vi "Exercise 7.1_Instant_Stop.vi"() -> ()   [LabVIEW 2020]
uses:
  7.1 States.ctl
panel:
  in  "Stop":bool
  out "Walk Sign":bool
  out "Green":bool
  out "Yellow":bool
  out "Red":bool
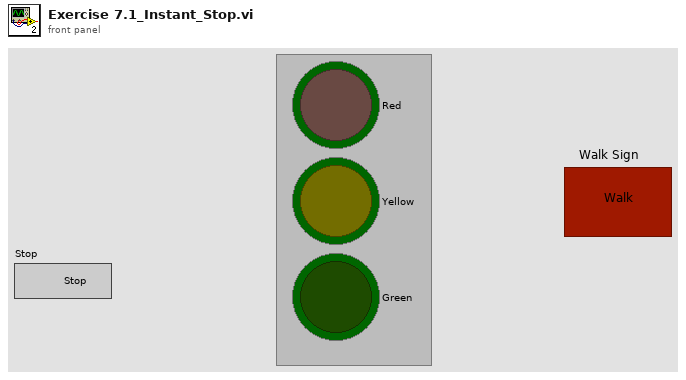
[diagram p1: front panel]
types:
  T1 = typedef "7.1 States.ctl" = enum16{"Initialize", "Green", "Yellow", "Red 1", "Red 2", "Stop"}
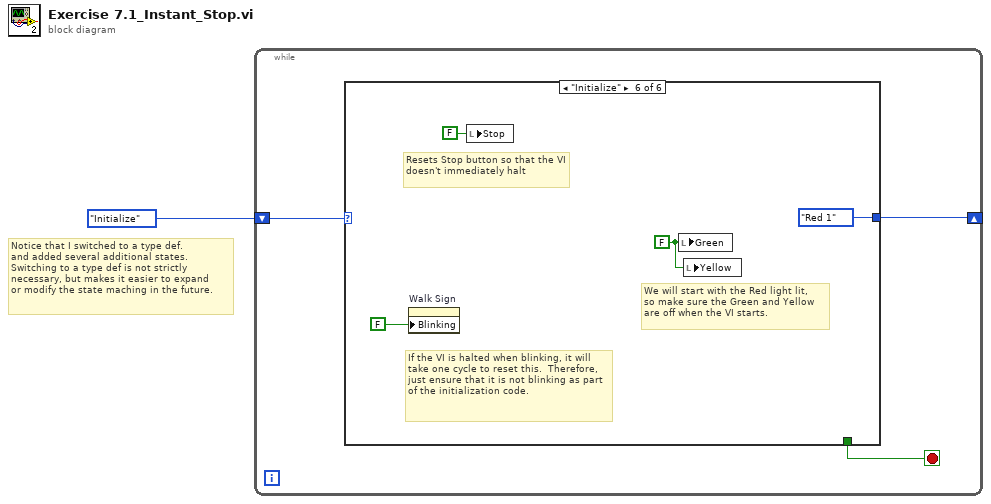
[diagram p0: block diagram]
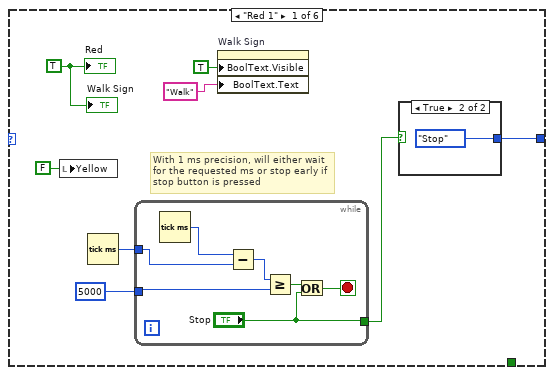
[diagram p2: hidden frame]
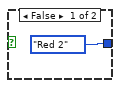
[diagram p3: hidden frame]
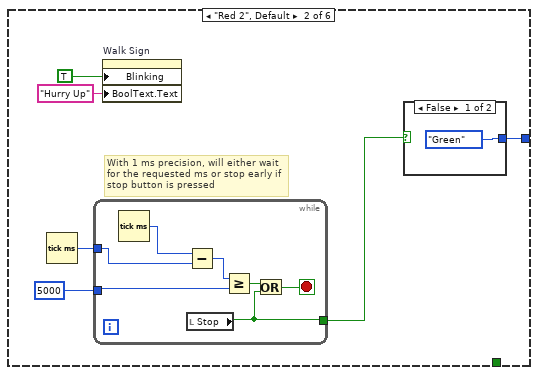
[diagram p4: hidden frame]
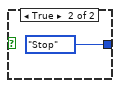
[diagram p5: hidden frame]
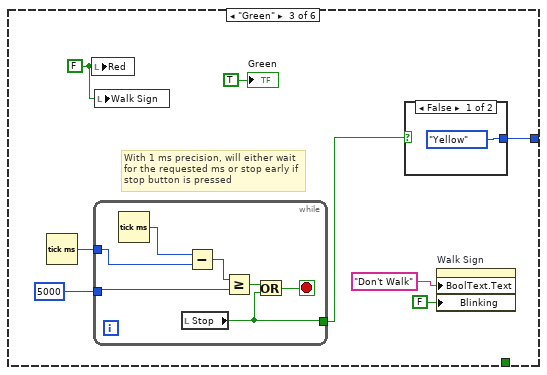
[diagram p6: hidden frame]
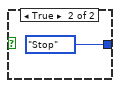
[diagram p7: hidden frame]
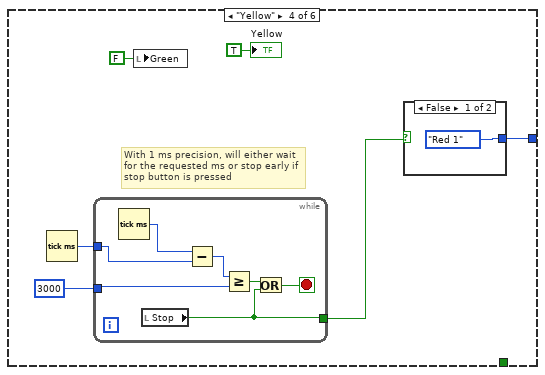
[diagram p8: hidden frame]
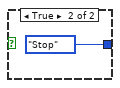
[diagram p9: hidden frame]
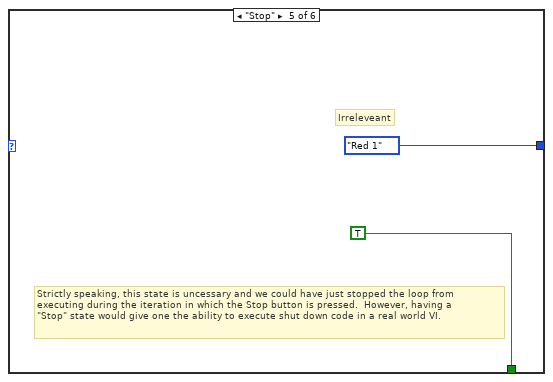
[diagram p10: hidden frame]
diagram:
  # "Notice that I switched to a type def.\nand added several additional states.\nSwitching to a type def is not strictly \nnecessary, but makes it easier to expand\nor modify the state maching in the future."
  n1 = while {
    shift-right: [w3] -> _
    shift-left: 7.1_States."Initialize" -> [w4]
    stop <- w2 stop-if-true
    n2 = case shown="\"Initialize\"" w4 {
      tunnel: [w9 w26 w41 w57 7.1_States."Red 1" 7.1_States."Red 1"] -> w3
      tunnel: [_ _ _ _ TRUE _] -> w2
      frame "Red 1" {
        w11 = TRUE ("Red")
        # "With 1 ms precision, will either wait for the requested ms or stop early if stop button is pressed"
        n3 = local write "Yellow"(FALSE ("Yellow")) -> ()
        n4 = Tick Count (ms)() -> (millisecond timer value=w7:u32)
        n5 = while {
          tunnel: w7 -> [w18]
          tunnel: u32 5000 ("milliseconds to wait") -> [w16]
          tunnel: ["Stop"] -> w5
          stop <- w14 stop-if-true
          n6 = Tick Count (ms)() -> (millisecond timer value=w19:u32)
          n7 = Subtract(x=w19, y=w18) -> (x-y=w17:u32)
          n8 = Greater Or Equal?(x=w17, y=w16) -> (x >= y?=w15:bool)
          n9 = Or(x=w15, y="Stop") -> (x .or. y?=w14:bool)
        }
        n10 = property on="Walk Sign" class="Bool"("BoolText.Visible"=TRUE ("Boolean Text.Visible"), "BoolText.Text"="Walk" ("Boolean Text.Text")) -> ()  [unwired: 2 in, 2 out]
        n11 = case shown="True" w5 {
          tunnel: [7.1_States."Red 2" 7.1_States."Stop"] -> w9
          frame False {
          }
          frame True {
          }
        }
        "Red" <- w11
        "Walk Sign" <- w11
      }
      frame "Red 2", Default {
        # "With 1 ms precision, will either wait for the requested ms or stop early if stop button is pressed"
        n12 = Tick Count (ms)() -> (millisecond timer value=w24:u32)
        n13 = while {
          tunnel: w24 -> [w33]
          tunnel: u32 5000 ("milliseconds to wait") -> [w31]
          tunnel: [w28] -> w22
          stop <- w29 stop-if-true
          n14 = Tick Count (ms)() -> (millisecond timer value=w34:u32)
          n15 = Subtract(x=w34, y=w33) -> (x-y=w32:u32)
          n16 = local read "Stop"() -> (w28:bool)
          n17 = Greater Or Equal?(x=w32, y=w31) -> (x >= y?=w30:bool)
          n18 = Or(x=w30, y=w28) -> (x .or. y?=w29:bool)
        }
        n19 = property on="Walk Sign" class="Bool"("Blinking"=TRUE, "BoolText.Text"="Hurry Up" ("Boolean Text.Text")) -> ()  [unwired: 2 in, 2 out]
        n20 = case shown="False" w22 {
          tunnel: [7.1_States."Green" 7.1_States."Stop"] -> w26
          frame False {
          }
          frame True {
          }
        }
      }
      frame "Green" {
        w44 = FALSE ("Red")
        # "With 1 ms precision, will either wait for the requested ms or stop early if stop button is pressed"
        n21 = Tick Count (ms)() -> (millisecond timer value=w39:u32)
        n22 = local write "Red"(w44) -> ()
        n23 = while {
          tunnel: w39 -> [w50]
          tunnel: u32 5000 ("milliseconds to wait") -> [w48]
          tunnel: [w45] -> w37
          stop <- w46 stop-if-true
          n24 = Tick Count (ms)() -> (millisecond timer value=w51:u32)
          n25 = local read "Stop"() -> (w45:bool)
          n26 = Subtract(x=w51, y=w50) -> (x-y=w49:u32)
          n27 = Greater Or Equal?(x=w49, y=w48) -> (x >= y?=w47:bool)
          n28 = Or(x=w47, y=w45) -> (x .or. y?=w46:bool)
        }
        n29 = local write "Walk Sign"(w44) -> ()
        n30 = case shown="False" w37 {
          tunnel: [7.1_States."Yellow" 7.1_States."Stop"] -> w41
          frame False {
          }
          frame True {
          }
        }
        n31 = property on="Walk Sign" class="Bool"("BoolText.Text"="Don't Walk" ("Boolean Text.Text"), "Blinking"=FALSE) -> ()  [unwired: 2 in, 2 out]
        "Green" <- TRUE ("Green")
      }
      frame "Yellow" {
        # "With 1 ms precision, will either wait for the requested ms or stop early if stop button is pressed"
        n32 = Tick Count (ms)() -> (millisecond timer value=w56:u32)
        n33 = while {
          tunnel: w56 -> [w65]
          tunnel: u32 3000 ("milliseconds to wait") -> [w63]
          tunnel: [w60] -> w54
          stop <- w61 stop-if-true
          n34 = Tick Count (ms)() -> (millisecond timer value=w66:u32)
          n35 = local read "Stop"() -> (w60:bool)
          n36 = Subtract(x=w66, y=w65) -> (x-y=w64:u32)
          n37 = Greater Or Equal?(x=w64, y=w63) -> (x >= y?=w62:bool)
          n38 = Or(x=w62, y=w60) -> (x .or. y?=w61:bool)
        }
        n39 = local write "Green"(FALSE ("Green")) -> ()
        n40 = case shown="False" w54 {
          tunnel: [7.1_States."Red 1" 7.1_States."Stop"] -> w57
          frame False {
          }
          frame True {
          }
        }
        "Yellow" <- TRUE ("Yellow")
      }
      frame "Stop" {
        # "Strictly speaking, this state is uncessary and we could have just stopped the loop from\nexecuting during the iteration in which the Stop button is pressed.  However, having a \n\"Stop\" state would give one the ability to execute shut down code in a real world VI."
        # "Irreleveant"
      }
      frame "Initialize" {
        w71 = FALSE ("Green")
        # "We will start with the Red light lit,\nso make sure the Green and Yellow\nare off when the VI starts."
        # "If the VI is halted when blinking, it will take one cycle to reset this.  Therefore, just ensure that it is not blinking as part of the initialization code."
        # "Resets Stop button so that the VI doesn't immediately halt"
        n41 = property on="Walk Sign" class="Bool"("Blinking"=FALSE) -> ()  [unwired: 2 in, 2 out]
        n42 = local write "Stop"(FALSE ("Stop")) -> ()
        n43 = local write "Green"(w71) -> ()
        n44 = local write "Yellow"(w71) -> ()
      }
    }
  }
